vi "createEntityJson.vi"(8 "error in (no error)":errorcluster, 10 "Data":T1={"ID"="", "Date"="2", "StreetAddress"="3", "longitude"="4", "latitude"="5", "Device"="6", "Index"=""}) -> (0 "error out":errorcluster, 2 "AirQualityObservedEntity":string)   [LabVIEW 2018]
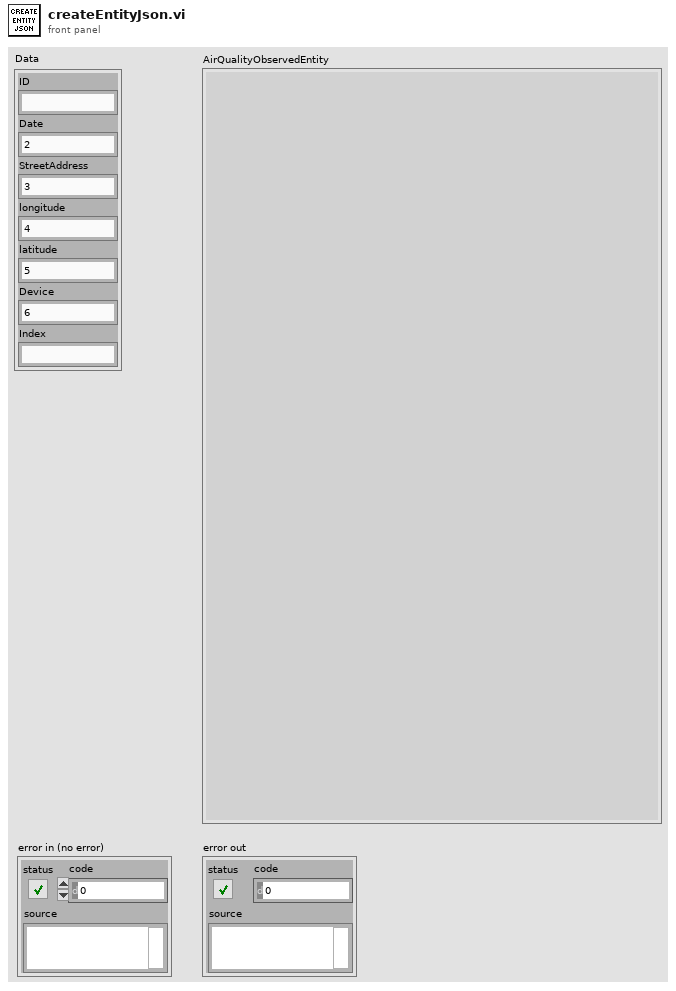
[diagram p1: front panel]
types:
  T1 = cluster{"ID":string, "Date":string, "StreetAddress":string, "longitude":string, "latitude":string, "Device":string, "Index":string}
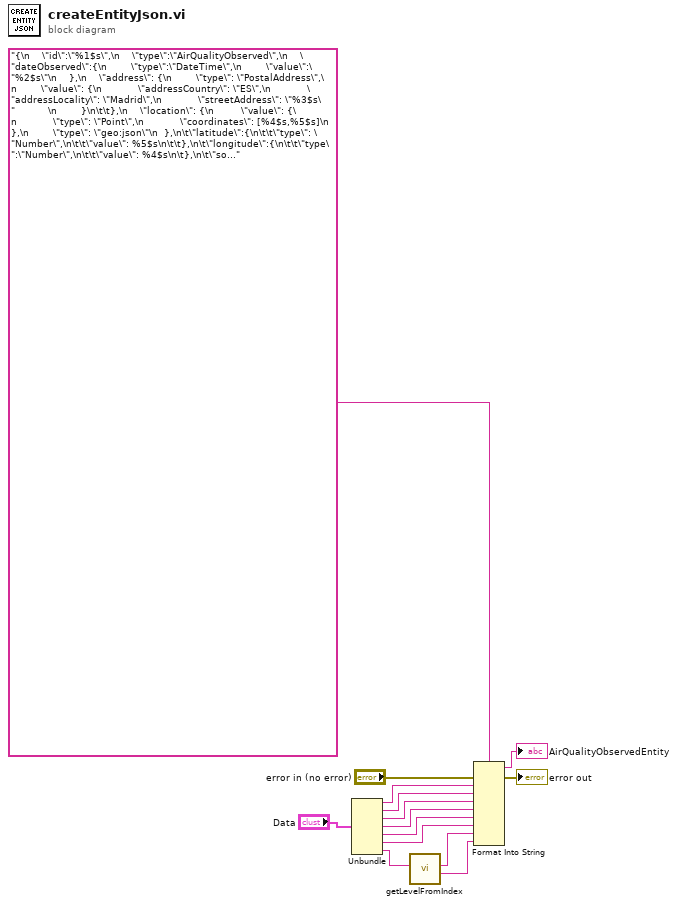
[diagram p0: block diagram]
diagram:
  n1 = Unbundle("Data") -> ("ID"=w9:string, "Date"=w8:string, "StreetAddress"=w7:string, "longitude"=w6:string, "latitude"=w5:string, "Device"=w4:string, "Index"=w3:string)
  n2 = call "getLevelFromIndex.vi"("Index"=w3) -> ("Level"=w1:string, "Index out"=w2:string)  [unwired: 9 in]
  n3 = Format Into String(format string="{\n    \"id\":\"%1$s\",\n    \"type\":\"AirQualityObserved\",\n    \"dateObserved\":{\n        \"type\":\"DateTime\",\n        \"value\":\"%2$s\"\n    },\n    \"address\": {\n        \"type\": \"PostalAddress\",\n        \"value\": {\n            \"addressCountry\": \"ES\",\n            \"addressLocality\": \"Madrid\",\n            \"streetAddress\": \"%3$s\"           \n        }\n\t\t},\n    \"location\": {\n         \"value\": {\n            \"type\": \"Point\",\n            \"coordinates\": [%4$s,%5$s]\n        },\n        \"type\": \"geo:json\"\n  },\n\t\"latitude\":{\n\t\t\"type\": \"Number\",\n\t\t\"value\": %5$s\n\t\t},\n\t\"longitude\":{\n\t\t\"type\":\"Number\",\n\t\t\"value\": %4$s\n\t},\n\t\"source\":{\n        \"type\":\"Text\",\n        \"value\":\"http://localhost:3000/d/mUqFaqaGk/airquality\"\n    },\n    \"airQualityLevel\":{\n        \"type\":\"Text\",\n        \"value\":\"%8$s\"\n    },\n\t    \"airQualityIndex\":{\n        \"type\":\"Number\",\n        \"value\":%7$s\n    },\n    \"refDevice\":{\n        \"type\":\"Relationship\",\n        \"value\":\"feather:%6$s\"\n    }\n}", error in="error in (no error)", w9, w8, w7, w6, w5, w4, w2, w1) -> (resulting string=→"AirQualityObservedEntity":string, error out=→"error out":errorcluster)  [unwired: 1 in]
